vi "SetEnableStateToTabCtrl.vi"(9 "페이지 활성화 상태":T1(ring), 10 "page index":i32=2, 11 "tab ctrl in":refnum<vi>) -> (3 "tab ctrl out":refnum<vi>)   [LabVIEW 2018, in "Library-Ctrl.lvlib"]
uses:
  Library-Ctrl.lvlib
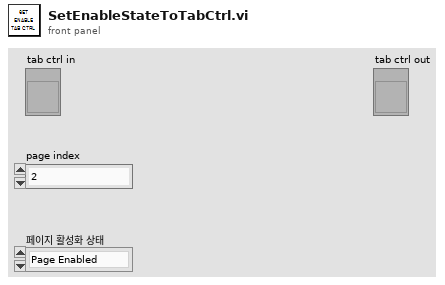
[diagram p1: front panel]
types:
  T1 = enum32{"Page Enabled", "Page Disabled", "Page Disabled & Grayed"}
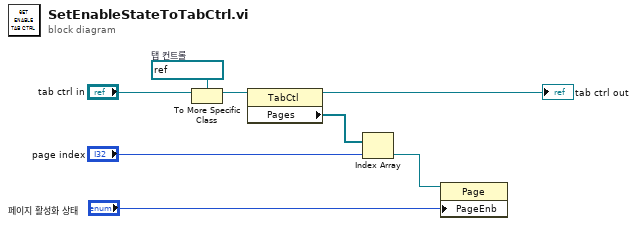
[diagram p0: block diagram]
diagram:
  w7 = refnum<vi> refnum  # 탭 컨트롤
  n1 = To More Specific Class(target class=w7, reference="tab ctrl in") -> (specific class reference=w6:refnum<vi>)  [unwired: 1 in, 1 out]
  n2 = property class="TabCtl"(reference=w6) -> (reference out=→"tab ctrl out":refnum<vi>, "Pages"=w5:refnum<vi>[])  [unwired: 1 in, 1 out]
  n3 = Index Array(array=w5, index="page index") -> (element=w3:refnum<vi>)
  n4 = property class="Page"(reference=w3, "PageEnb"="페이지 활성화 상태") -> ()  [unwired: 1 in, 2 out]
